vi "StringConcatenate.vi"() -> ()   [LabVIEW 2019]
panel:
  out "concatenated string":string
  in  "String 2":string
  in  "String":string
  out "String3":string
  in  "String2":string="World"
  in  "String1":string="Hello"
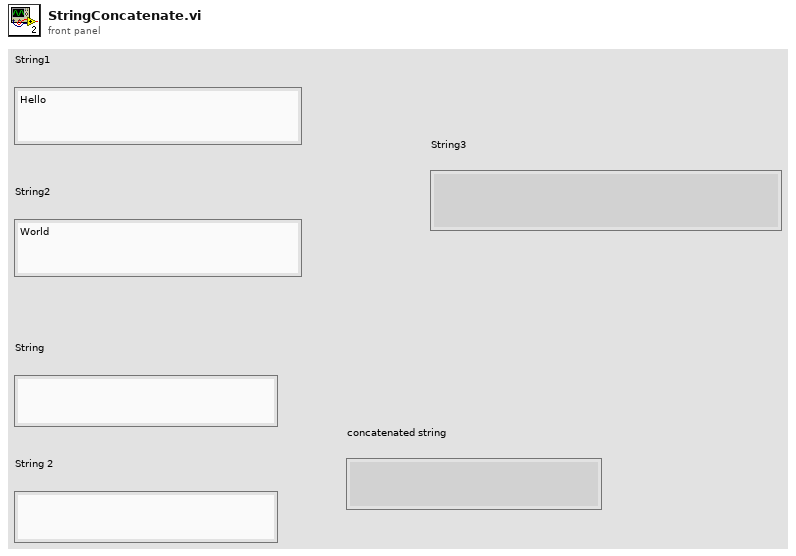
[diagram p1: front panel]
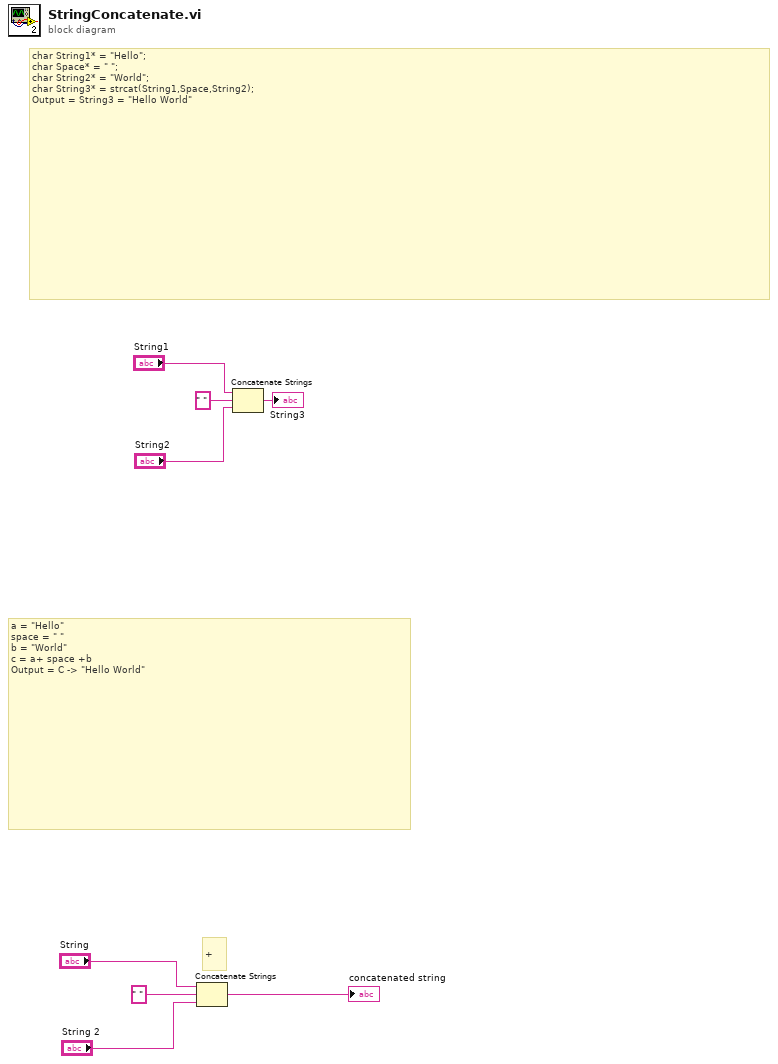
[diagram p0: block diagram]
diagram:
  # "+"
  # "a = \"Hello\"\nspace = \" \"\nb = \"World\"\nc = a+ space +b\nOutput = C -> \"Hello World\""
  # "char String1* = \"Hello\";\nchar Space* = \" \";\nchar String2* = \"World\";\nchar String3* = strcat(String1,Space,String2);\nOutput = String3 = \"Hello World\""
  n1 = Concatenate Strings("String", " " ("string"), "String 2") -> (→"concatenated string":string)
  n2 = Concatenate Strings("String1", " " ("string"), "String2") -> (→"String3":string)
